vi "Commit Excuse Note.vi"(8 "error in (no error)":errorcluster, 10 "ExcuseNote":T1, 11 "ExcuseNote in":refnum<class "ExcuseNote.lvclass">) -> (0 "error out":errorcluster, 3 "ExcuseNote out":refnum<class "ExcuseNote.lvclass">)   [LabVIEW 2015, in "ExcuseNote.lvclass"]
uses:
  ExcuseNote.lvclass
  ExcuseNote.lvclass/ExcuseNote.ctl
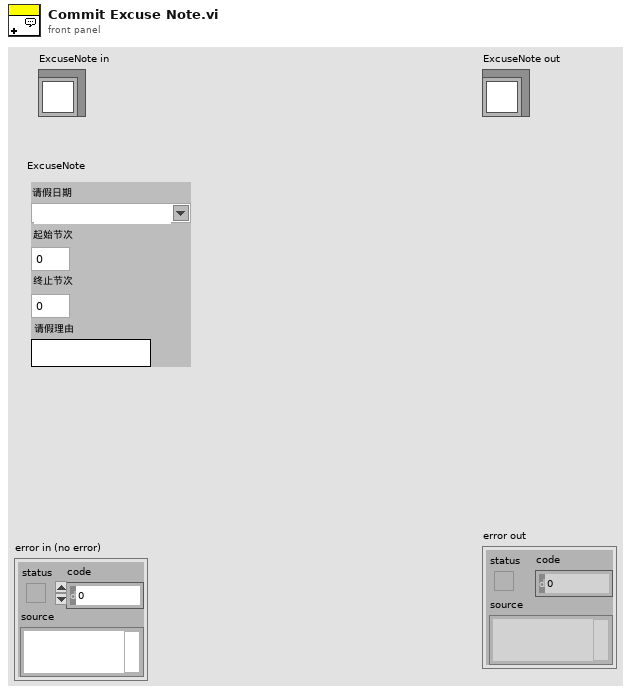
[diagram p1: front panel]
types:
  T1 = cluster{"请假日期":string, "起始节次":i32, "终止节次":i32, "请假理由":string}
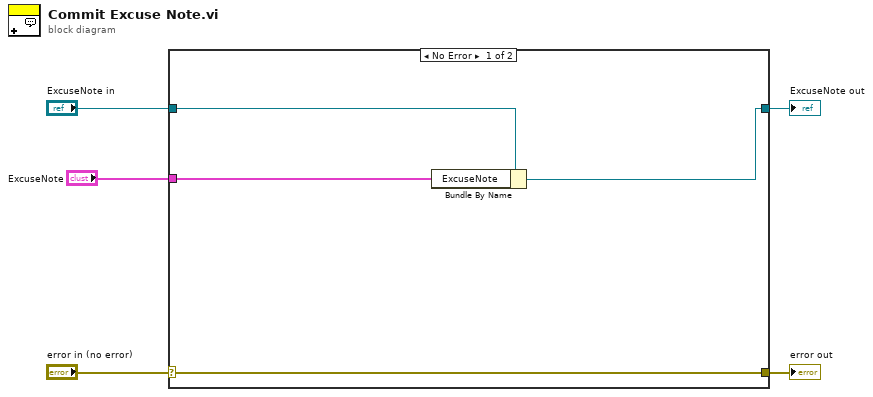
[diagram p0: block diagram]
diagram:
  n1 = case shown="No Error" "error in (no error)" {
    selector: "error in (no error)" -> [w9 w11]
    tunnel: [w9 w11] -> w4
    tunnel: [w7 w10] -> w2
    tunnel: "ExcuseNote in" -> [w8 w10]
    tunnel: "ExcuseNote" -> [w6 _]
    frame No Error {
      n2 = Bundle By Name(cluster=w8, "ExcuseNote"=w6) -> (w7:refnum<class "ExcuseNote.lvclass">)
    }
    frame Error {
    }
  }
  "error out" <- w4
  "ExcuseNote out" <- w2
